vi "LBCB Number 2 Source Text.vi"(10 "Combined":bool, 11 "LBCB Number":T1) -> (3 "Source String":string)   [LabVIEW 2013]
uses:
  Data Access Objects/Metadata/LBCB Number.ctl
  Names/Source Group Type.ctl
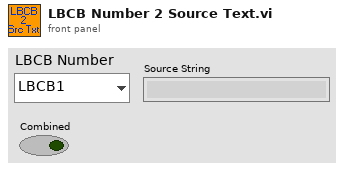
[diagram p1: front panel]
types:
  T1 = typedef "LBCB Number.ctl" = enum16{"LBCB1", "LBCB2"}
  T2 = typedef "Source Group Type.ctl" = enum16{"LBCB1", "LBCB2", "Consolidated", "External"}
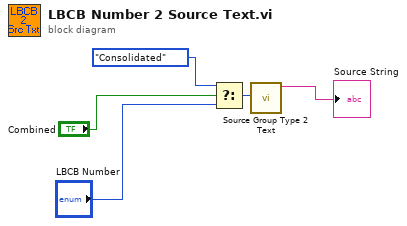
[diagram p0: block diagram]
diagram:
  n1 = Select(t=Source_Group_Type."Consolidated" ("Source Group"), s="Combined", f="LBCB Number") -> (s? t:f=w2:T2)
  n2 = call "Source Group Type 2 Text.vi"("Source"=w2) -> ("String"=→"Source String":string)  [unwired: 10 in]
